vi "GRAB_MOVE.vi"(6 "ARM 2 FEEDBACK":dbl, 7 "RESET":bool, 8 "ARM 1 FEEDBACK":dbl, 9 "ARM 2 INITIAL IN":dbl, 10 "ARM 1 INITIAL":dbl, 11 "INPUT":bool) -> (0 "ARM 2 SETPOINT OUT":dbl, 2 "RUNNING?":bool, 3 "ARM 1 SETPOINT OUT":dbl)   [LabVIEW 2017]
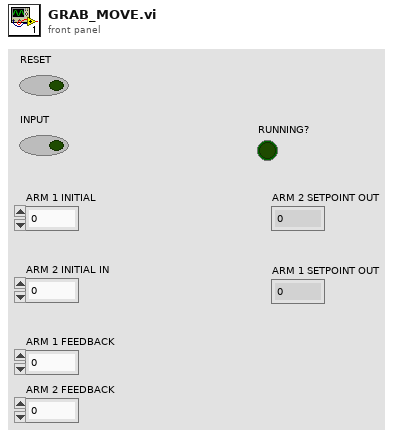
[diagram p1: front panel]
types:
  T1 = enum16{"START", "STEP 1", "STEP 2", "STEP 3", "STEP 4"}
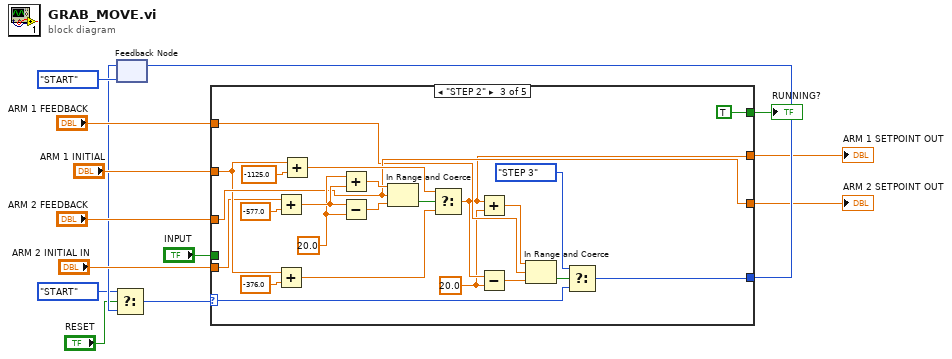
[diagram p0: block diagram]
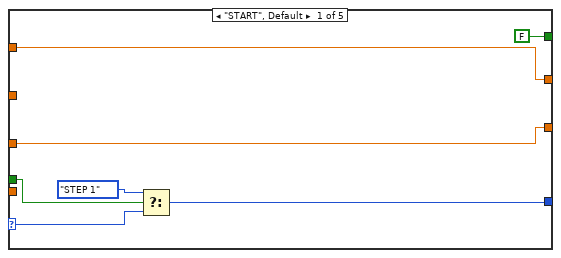
[diagram p2: hidden frame]
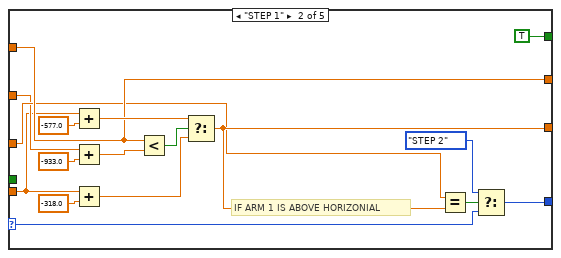
[diagram p3: hidden frame]
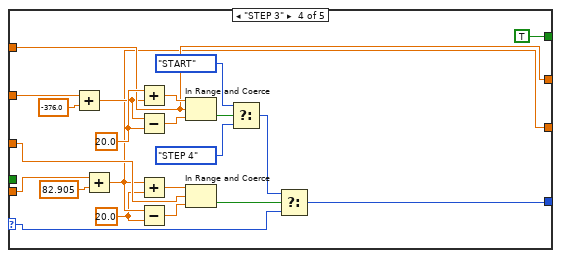
[diagram p4: hidden frame]
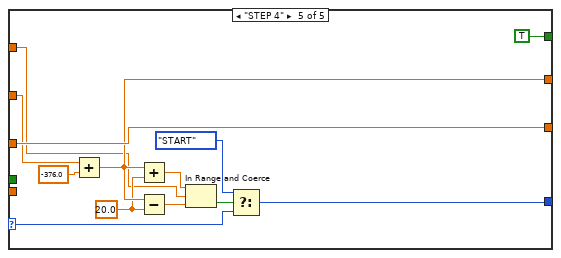
[diagram p5: hidden frame]
diagram:
  n1 = feedback #1(T1."START" ("t")) -> (w4:T1)
  n2 = Select(t=T1."START", s="RESET", f=w4) -> (s? t:f=w3:T1)
  n3 = case shown="\"STEP 2\"" w3 {
    selector: w3 -> [w20 w38 w61 w83 w96]
    tunnel: [w21 w37 w60 w82 w95] -> w14
    tunnel: "INPUT" -> [w16 _ _ _ _]
    tunnel: "ARM 1 INITIAL" -> [_ w23 w40 w71 w90]
    tunnel: "ARM 2 INITIAL IN" -> [_ w22 w39 w68 _]
    tunnel: "ARM 2 FEEDBACK" -> [w18 w25 w50 w67 w92]
    tunnel: [w18 w28 w50 w64 w92] -> w9
    tunnel: "ARM 1 FEEDBACK" -> [w19 w29 w47 w77 w84]
    tunnel: [w19 w29 w44 w77 w86] -> w7
    tunnel: [FALSE TRUE TRUE TRUE TRUE] -> w6
    frame "START", Default {
      n4 = Select(t=T1."STEP 1", s=w16, f=w20) -> (s? t:f=w21:T1)
    }
    frame "STEP 1" {
      # "IF ARM 1 IS ABOVE HORIZONIAL"
      n5 = Add(x=w22, y=-577.0) -> (x+y=w33:dbl)
      n6 = Add(x=w23, y=-933.0) -> (x+y=w31:dbl)
      n7 = Add(x=w22, y=-318.0) -> (x+y=w27:dbl)
      n8 = Less?(x=w29, y=w31) -> (x < y?=w34:bool)
      n9 = Select(t=w33, s=w34, f=w27) -> (s? t:f=w28:dbl)
      n10 = Equal?(x=w25, y=w28) -> (x = y?=w36:bool)
      n11 = Select(t=T1."STEP 2", s=w36, f=w38) -> (s? t:f=w37:T1)
    }
    frame "STEP 2" {
      w43 = 20.0 ("y")
      w54 = 20.0 ("x")
      n12 = Add(x=w39, y=-577.0) -> (x+y=w55:dbl)
      n13 = Add(x=w40, y=-376.0) -> (x+y=w41:dbl)
      n14 = Add(x=w40, y=-1125.0) -> (x+y=w52:dbl)
      n15 = Add(x=w54, y=w55) -> (x+y=w57:dbl)
      n16 = Subtract(x=w55, y=w54) -> (x-y=w56:dbl)
      n17 = In Range and Coerce(upper limit=w57, x=w50, lower limit=w56) -> (In Range?=w53:bool)  [unwired: 1 out]
      n18 = Select(t=w52, s=w53, f=w41) -> (s? t:f=w44:dbl)
      n19 = Add(x=w44, y=w43) -> (x+y=w46:dbl)
      n20 = Subtract(x=w44, y=w43) -> (x-y=w45:dbl)
      n21 = In Range and Coerce(upper limit=w46, x=w47, lower limit=w45) -> (In Range?=w48:bool)  [unwired: 1 out]
      n22 = Select(t=T1."STEP 3", s=w48, f=w61) -> (s? t:f=w60:T1)
    }
    frame "STEP 3" {
      w63 = 20.0 ("y")
      w78 = 20.0 ("x")
      n23 = Add(x=w71, y=-376.0) -> (x+y=w70:dbl)
      n24 = Add(x=w68, y=82.905) -> (x+y=w64:dbl)
      n25 = Add(x=w78, y=w70) -> (x+y=w80:dbl)
      n26 = Subtract(x=w70, y=w78) -> (x-y=w79:dbl)
      n27 = Add(x=w64, y=w63) -> (x+y=w66:dbl)
      n28 = Subtract(x=w64, y=w63) -> (x-y=w65:dbl)
      n29 = In Range and Coerce(upper limit=w80, x=w77, lower limit=w79) -> (In Range?=w73:bool)  [unwired: 1 out]
      n30 = In Range and Coerce(upper limit=w66, x=w67, lower limit=w65) -> (In Range?=w62:bool)  [unwired: 1 out]
      n31 = Select(t=T1."START", s=w73, f=T1."STEP 4" ("t")) -> (s? t:f=w76:T1)
      n32 = Select(t=w76, s=w62, f=w83) -> (s? t:f=w82:T1)
    }
    frame "STEP 4" {
      w85 = 20.0 ("y")
      n33 = Add(x=w90, y=-376.0) -> (x+y=w86:dbl)
      n34 = Add(x=w86, y=w85) -> (x+y=w88:dbl)
      n35 = Subtract(x=w86, y=w85) -> (x-y=w87:dbl)
      n36 = In Range and Coerce(upper limit=w88, x=w84, lower limit=w87) -> (In Range?=w89:bool)  [unwired: 1 out]
      n37 = Select(t=T1."START", s=w89, f=w96) -> (s? t:f=w95:T1)
    }
  }
  "ARM 2 SETPOINT OUT" <- w9
  "ARM 1 SETPOINT OUT" <- w7
  "RUNNING?" <- w6
  n38 = feedback-in #1(w14) -> ()
